vi "Square wave.vi"(5 "Low":i32=50, 7 "High":i32=50, 8 "error in (no error)":errorcluster, 10 "Amplitude":i32=100, 11 "Length (steps)":i32=30) -> (0 "error out":errorcluster)   [LabVIEW 2017]
doc: "To draw a square wave around the spherical object."
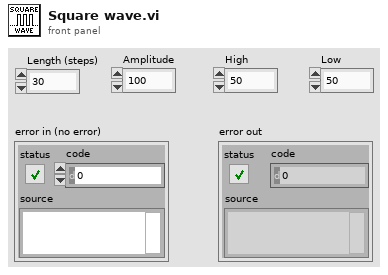
[diagram p1: front panel]
types:
  T1 = enum16{"Full", "Half", "Quarter", "Eighth", "Sixteenth"}
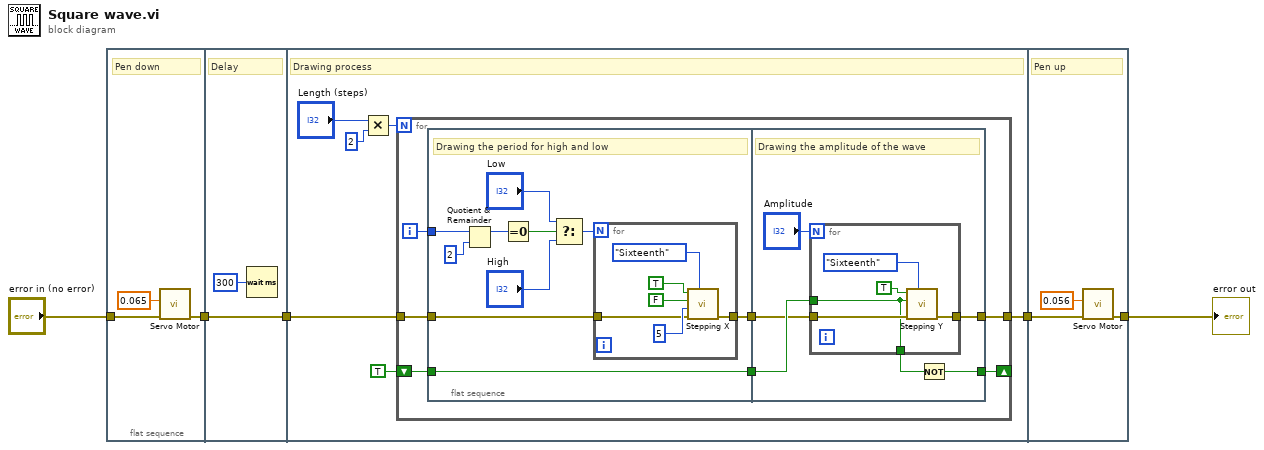
[diagram p0: block diagram]
diagram:
  n1 = flat-sequence {
    tunnel: [w7] -> w2
    tunnel: "error in (no error)" -> [w6]
    tunnel: w2 -> [w10]
    tunnel: [w10] -> w1
    tunnel: w1 -> [w12]
    tunnel: [w11] -> w5
    tunnel: w5 -> [w52]
    tunnel: [w51] -> w4
    frame #0 {
      # "Pen down"
      n2 = call "Servo Motor.vi"("error in (no error)"=w6, "Duty Cycle"=0.065) -> ("error out"=w7:errorcluster)  [unwired: 9 in]
    }
    frame #1 {
      # "Delay"
      n3 = Wait (ms)(milliseconds to wait=u32 300) -> ()  [unwired: 1 out]
    }
    frame #2 {
      # "Drawing process"
      n4 = Multiply(x="Length (steps)", y=2) -> (x*y=w14:i32)
      n5 = for {
        N: w14 -> [_]
        shift-right: [w21] -> _
        shift-left: TRUE -> [w22]
        tunnel: w12 -> [w19]
        tunnel: [w18] -> w11
        i -> [w17]
        n6 = flat-sequence {
          tunnel: [w33] -> w23
          tunnel: w22 -> [w33]
          tunnel: [w32] -> w20
          tunnel: w19 -> [w31]
          tunnel: w17 -> [w30]
          tunnel: w23 -> [w44]
          tunnel: [w42] -> w21
          tunnel: w20 -> [w41]
          tunnel: [w40] -> w18
          frame #0 {
            # "Drawing the period for high and low"
            n7 = Quotient & Remainder(x=w30, y=2) -> (x-y*floor(x/y)=w28:i32)  [unwired: 1 out]
            n8 = Equal To 0?(x=w28) -> (x = 0?=w27:bool)
            n9 = Select(t="Low", s=w27, f="High") -> (s? t:f=w24:i32)
            n10 = for {
              N: w24 -> [_]
              tunnel: [w39] -> w32
              tunnel: w31 -> [w34]
              n11 = call "Stepping X.vi"("Microstep size"=T1."Sixteenth", "error in (no error)"=w34, "Delay"=u32 5 ("Speed"), "Direction"=FALSE, "Enable"=TRUE) -> ("error out"=w39:errorcluster)  [unwired: 6 in]
            }
          }
          frame #1 {
            # "Drawing the amplitude of the wave"
            n12 = for {
              N: "Amplitude" -> [_]
              tunnel: w44 -> [w47]
              tunnel: [w47] -> w43
              tunnel: w41 -> [w50]
              tunnel: [w46] -> w40
              n13 = call "Stepping Y.vi"("Microstep size"=T1."Sixteenth", "error in (no error)"=w50, "Direction"=w47, "Enable"=TRUE) -> ("error out"=w46:errorcluster)  [unwired: 7 in]
            }
            n14 = Not(x=w43) -> (.not. x?=w42:bool)
          }
        }
      }
    }
    frame #3 {
      # "Pen up"
      n15 = call "Servo Motor.vi"("error in (no error)"=w52, "Duty Cycle"=0.056) -> ("error out"=w51:errorcluster)  [unwired: 9 in]
    }
  }
  "error out" <- w4
